vi "Send Set Vehicle Position from wash step.vi"(7 "Message Priority (Normal)":T2=enum."Normal", 8 "error in (no error)":errorcluster, 10 "Car Wash Steps":T1, 11 "Message Enqueuer":refnum<class "Message Enqueuer.lvclass">) -> (0 "error out":errorcluster, 3 "Message Enqueuer out":refnum<class "Message Enqueuer.lvclass">)   [LabVIEW 2019, in "Car Wash Controller Actor.lvlib" / "Set Vehicle Position from wash step Msg.lvclass"]
doc: "This VI sends the message to an actor."
uses:
  Set Vehicle Position from wash step Msg.lvclass
  <vilib>/ActorFramework/Message Enqueuer/Message Enqueuer.lvclass
  <vilib>/ActorFramework/Message Enqueuer/Message Priority.ctl
  Sim Entry Console Actor/Sim Entry Console Actor/Wash steps selection -Buttons.ctl
  C:/Program Files (x86)/National Instruments/LabVIEW 2019/vi.lib/ActorFramework/Message/Message.lvclass
  Set Vehicle Position from wash step Msg.lvclass/Set Vehicle Position from wash step Msg.ctl
  <vilib>/ActorFramework/Message Enqueuer/Message Enqueuer.lvclass/Message Enqueuer.ctl
  <vilib>/ActorFramework/Message Priority Queue/Priority Enqueue.vi
  Sim Entry Console Actor/Sim Entry Console Actor/Simulated Entry Console Actor.lvclass
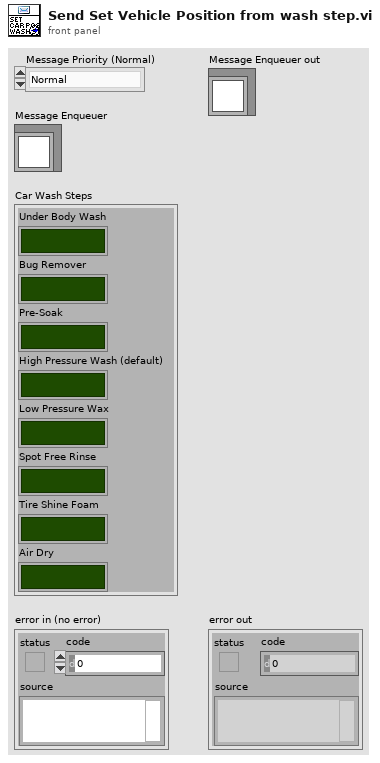
[diagram p1: front panel]
types:
  T1 = typedef "Simulated Entry Console Actor.lvlib/Simulated Entry Console Actor.lvclass/Wash steps selection -Buttons.ctl" = cluster{"Under Body Wash":bool, "Bug Remover":bool, "Pre-Soak":bool, "High Pressure Wash (default)":bool, "Low Pressure Wax":bool, "Spot Free Rinse":bool, "Tire Shine Foam":bool, "Air Dry":bool}
  T2 = typedef "Actor Framework.lvlib/Message Enqueuer.lvclass/Message Priority.ctl" = enum16{"Low", "Normal", "High"}
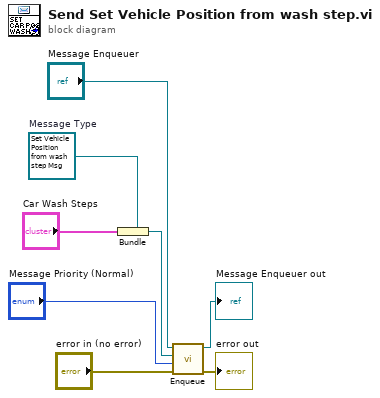
[diagram p0: block diagram]
diagram:
  w5 = refnum<class "Set Vehicle Position from wash step Msg.lvclass"> refnum  # Message Type
  n1 = Bundle(cluster=w5, "Car Wash Steps") -> (w4:refnum<class "Set Vehicle Position from wash step Msg.lvclass">)
  n2 = call <vilib>:"Enqueue.vi"("error in (no error)"="error in (no error)", "Message Priority (Normal)"="Message Priority (Normal)", "Message"=w4, "Message Enqueuer in"="Message Enqueuer") -> ("error out"=→"error out":errorcluster, "Message Enqueuer out"=→"Message Enqueuer out":refnum<class "Message Enqueuer.lvclass">)  [unwired: 6 in]
